vi "组合按键.vi"(8 "按键编号":string, 9 "动作":string(combo), 10 "按键名字":string(combo), 11 "面板地址":string(combo)) -> (3 "按键":T1)   [LabVIEW 2019]
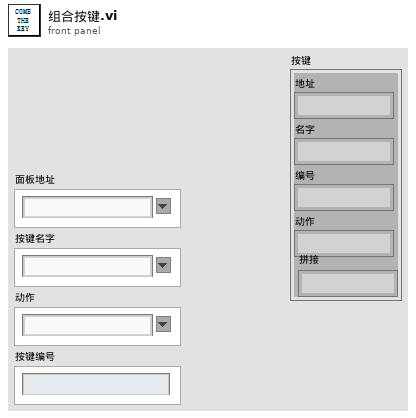
[diagram p1: front panel]
types:
  T1 = cluster{"地址":string, "名字":string, "编号":string, "动作":string, "拼接":string}
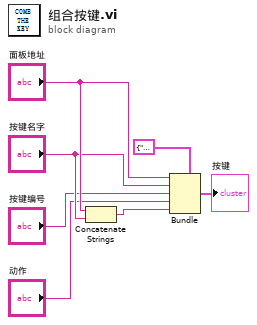
[diagram p0: block diagram]
diagram:
  n1 = Concatenate Strings("面板地址", "按键名字") -> (w6:string)
  n2 = Bundle(cluster=T1 {"地址"="", "名字"="", "编号"="", "动作"="", "拼接"=""} ("按键"), "地址"="面板地址", "名字"="按键名字", "编号"="按键编号", "动作"="动作", "拼接"=w6) -> (→"按键":T1)
